vi "UpdateResultElement.vi"(8 "Data":string, 9 "Lookup String":string, 10 "Report Header Indicies in":string[][](array[string]), 11 "Result in":string[][](array[string])) -> (2 "Report Header Indicies out":string[][](array[string]), 3 "Result Out":string[][](array[string]))   [LabVIEW 2015, in "csv-formatter.lvclass"]
uses:
  csv-formatter.lvclass
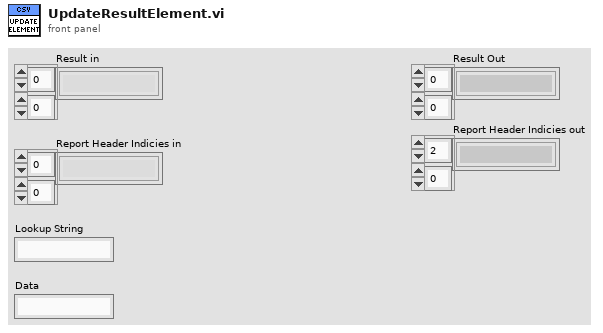
[diagram p1: front panel]
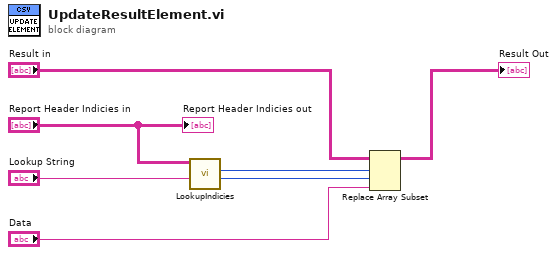
[diagram p0: block diagram]
diagram:
  n1 = call "LookupIndicies.vi"("Lookup String"="Lookup String", "Report Header Indicies"="Report Header Indicies in") -> ("Column"=w6:i32, "Row"=w5:i32)  [unwired: 8 in]
  n2 = Replace Array Subset(array="Result in", new element="Data", index (row)=w5, index (col)=w6) -> (→"Result Out":string[][])
  "Report Header Indicies out" <- "Report Header Indicies in"
